vi "ArmGetStatus.vi"(0 "Pivot Ref":T1={"DeviceStatus"={"status"=FALSE, "code"=0, "source"=""}, "Type"=enum."PWM", "PWM"={"PWM Channel"=enum."PWM 1", "DeadBand"={"Name"="", "maxPositivePwm"=0, "minPositivePwm"=0, "centerPwm"=0, "maxNegativePwm"=0, "minNegativePwm"=0, "angularRange"=0}}, "CAN"={"Device Number"=0, "Control Mode"=enum."Percent VBus", "Semaphore"=refnum, "Max Vout"=12.0, "TalonSRX Control Mode"=enum."Percent VBus"}, "Invert"=FALSE, "TransformRef"=refnum, "InvTransformRef"=refnum}, 5 "ExtensionRef":T1={"DeviceStatus"={"status"=FALSE, "code"=0, "source"=""}, "Type"=enum."PWM", "PWM"={"PWM Channel"=enum."PWM 1", "DeadBand"={"Name"="", "maxPositivePwm"=0, "minPositivePwm"=0, "centerPwm"=0, "maxNegativePwm"=0, "minNegativePwm"=0, "angularRange"=0}}, "CAN"={"Device Number"=0, "Control Mode"=enum."Percent VBus", "Semaphore"=refnum, "Max Vout"=12.0, "TalonSRX Control Mode"=enum."Percent VBus"}, "Invert"=FALSE, "TransformRef"=refnum, "InvTransformRef"=refnum}, 7 "Wrist Ref":T1={"DeviceStatus"={"status"=FALSE, "code"=0, "source"=""}, "Type"=enum."PWM", "PWM"={"PWM Channel"=enum."PWM 1", "DeadBand"={"Name"="", "maxPositivePwm"=0, "minPositivePwm"=0, "centerPwm"=0, "maxNegativePwm"=0, "minNegativePwm"=0, "angularRange"=0}}, "CAN"={"Device Number"=0, "Control Mode"=enum."Percent VBus", "Semaphore"=refnum, "Max Vout"=12.0, "TalonSRX Control Mode"=enum."Percent VBus"}, "Invert"=FALSE, "TransformRef"=refnum, "InvTransformRef"=refnum}, 11 "error in (no error)":errorcluster) -> (1 "Pivot Ref out":T1={"DeviceStatus"={"status"=FALSE, "code"=0, "source"=""}, "Type"=enum."PWM", "PWM"={"PWM Channel"=enum."Invalid", "DeadBand"={"Name"="", "maxPositivePwm"=0, "minPositivePwm"=0, "centerPwm"=0, "maxNegativePwm"=0, "minNegativePwm"=0, "angularRange"=0}}, "CAN"={"Device Number"=0, "Control Mode"=enum."Percent VBus", "Semaphore"=refnum, "Max Vout"=12.0, "TalonSRX Control Mode"=enum."Percent VBus"}, "Invert"=FALSE, "TransformRef"=refnum, "InvTransformRef"=refnum}, 2 "Extension Ref out":T1={"DeviceStatus"={"status"=FALSE, "code"=0, "source"=""}, "Type"=enum."PWM", "PWM"={"PWM Channel"=enum."Invalid", "DeadBand"={"Name"="", "maxPositivePwm"=0, "minPositivePwm"=0, "centerPwm"=0, "maxNegativePwm"=0, "minNegativePwm"=0, "angularRange"=0}}, "CAN"={"Device Number"=0, "Control Mode"=enum."Percent VBus", "Semaphore"=refnum, "Max Vout"=12.0, "TalonSRX Control Mode"=enum."Percent VBus"}, "Invert"=FALSE, "TransformRef"=refnum, "InvTransformRef"=refnum}, 3 "Wrist Ref out":T1={"DeviceStatus"={"status"=FALSE, "code"=0, "source"=""}, "Type"=enum."PWM", "PWM"={"PWM Channel"=enum."Invalid", "DeadBand"={"Name"="", "maxPositivePwm"=0, "minPositivePwm"=0, "centerPwm"=0, "maxNegativePwm"=0, "minNegativePwm"=0, "angularRange"=0}}, "CAN"={"Device Number"=0, "Control Mode"=enum."Percent VBus", "Semaphore"=refnum, "Max Vout"=12.0, "TalonSRX Control Mode"=enum."Percent VBus"}, "Invert"=FALSE, "TransformRef"=refnum, "InvTransformRef"=refnum}, 4 "Pivot angle (rad)":dbl(knob) scale=3.1416..-3.1416, 6 "Extension (in.)":dbl, 8 "Wrist angle (rad, relative to ground)":dbl(knob) scale=3.1416..-3.1416, 12 "Wrist X":dbl, 14 "Wrist Y":dbl, 15 "error out":errorcluster)   [LabVIEW 2015]
uses:
  <vilib>/Rock Robotics/WPI/MotorControl/WPI_MotorControlDeviceRef.ctl
  <vilib>/Rock Robotics/WPI/MotorControl/WPI_MotorControlType.ctl
  <vilib>/Rock Robotics/SystemInterfaces/DIO/FPGA_DIOPWMChannel.ctl
  <vilib>/Rock Robotics/WPI/PWM/WPI_PWMDeadband.ctl
  <vilib>/Rock Robotics/WPI/CAN/Jaguar/SubVIs/WPI_CANJaguar_ControlMode.ctl
  <vilib>/Rock Robotics/WPI/CAN/TalonSRX/WPI_CANTalonSRX_APIControlMode.ctl
  <vilib>/Rock Robotics/WPI/PWM/WPI_PWMTransform_ConPane.ctl
  Robot Global Data.vi
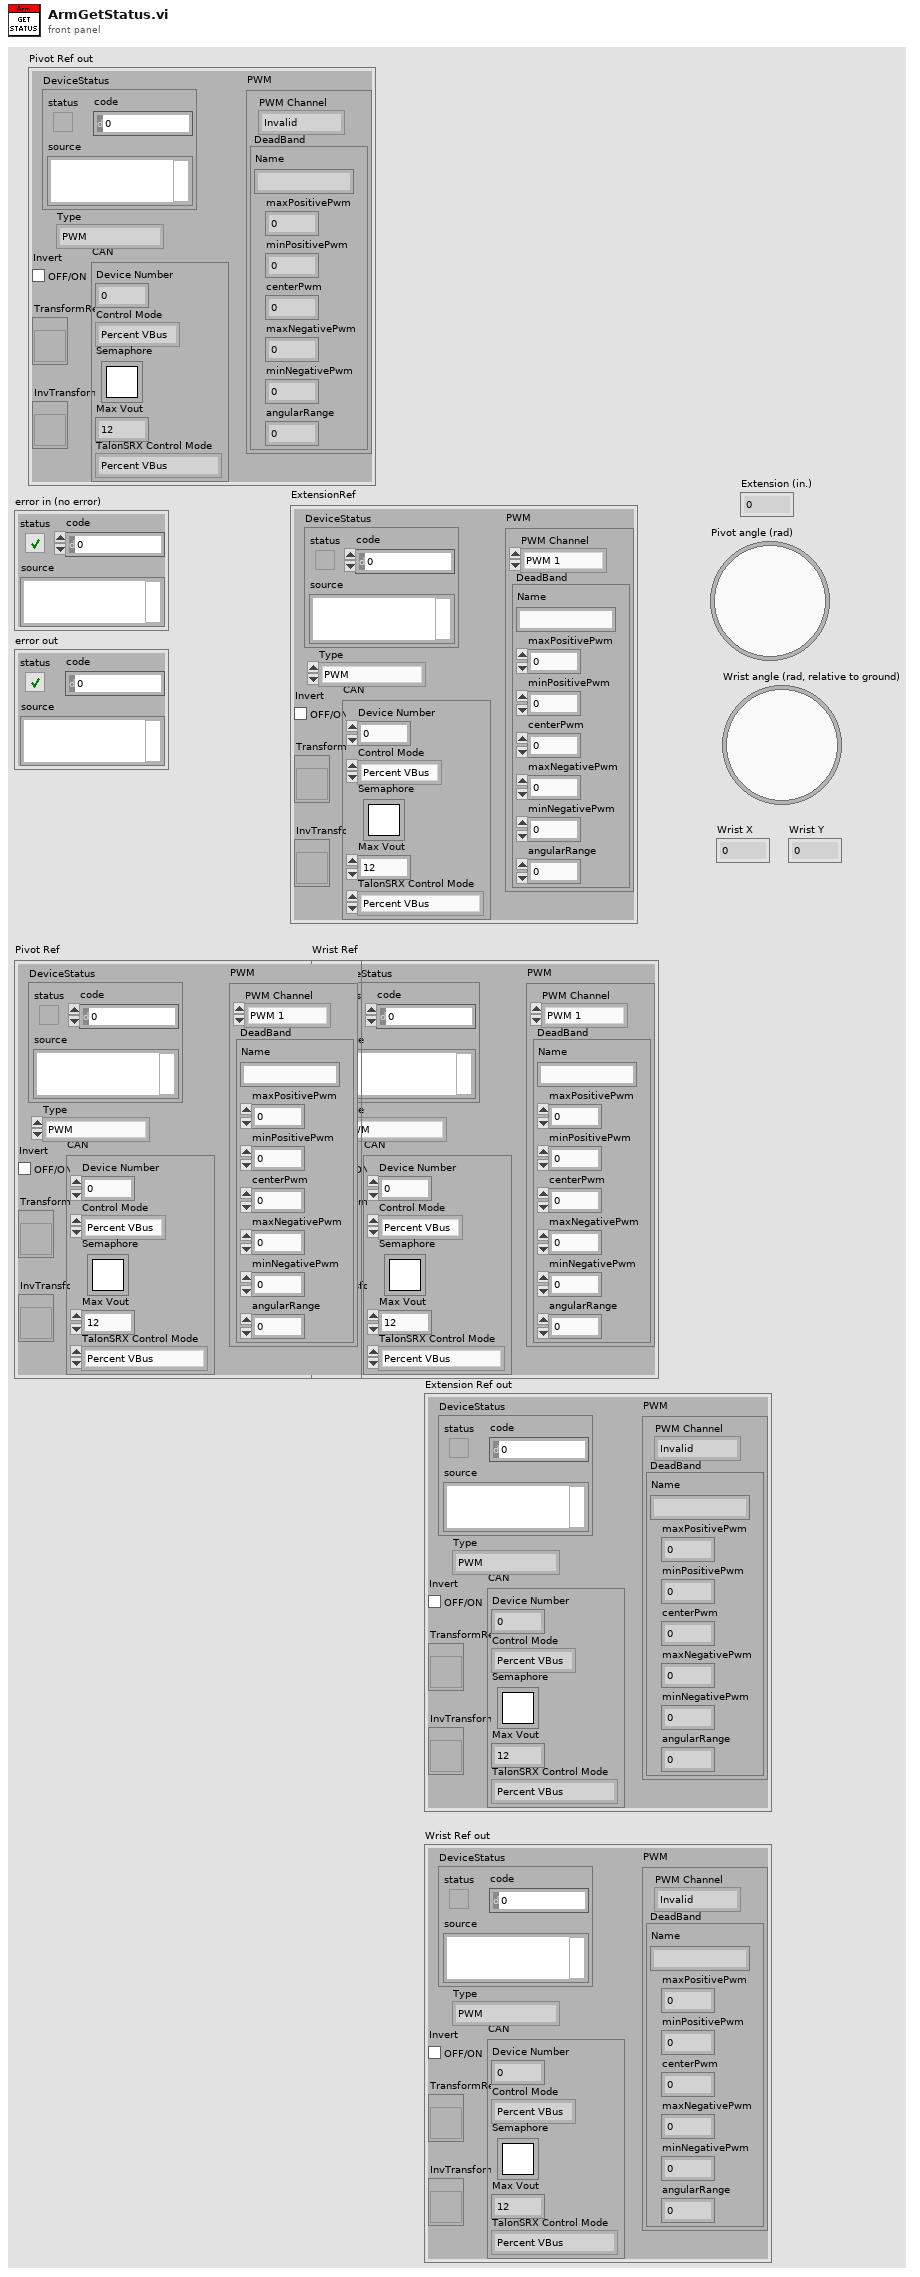
[diagram p1: front panel]
types:
  T1 = typedef "WPI_MotorControlDeviceRef.ctl" = cluster{"DeviceStatus":errorcluster, "Type":T2, "PWM":cluster{"PWM Channel":T3, "DeadBand":T4}, "CAN":cluster{"Device Number":u8, "Control Mode":T5, "Semaphore":T6, "Max Vout":dbl, "TalonSRX Control Mode":T7}, "Invert":bool, "TransformRef":T8, "InvTransformRef":T8}
  T2 = typedef "WPI_MotorControlType.ctl" = enum16{"PWM", "CAN", "CANTalonSRX"}
  T3 = typedef "FPGA_DIOPWMChannel.ctl" = enum8{"PWM 0", "PWM 1", "PWM 2", "PWM 3", "PWM 4", "PWM 5", "PWM 6", "PWM 7", "PWM 8", "PWM 9", "PWM MXP 0", "PWM MXP 1", "PWM MXP 2", "PWM MXP 3", "PWM MXP 4", "PWM MXP 5", "PWM MXP 6", "PWM MXP 7", "PWM MXP 8", "PWM MXP 9", "Invalid"}
  T4 = typedef "WPI_PWMDeadband.ctl" = cluster{"Name":string, "maxPositivePwm":i32, "minPositivePwm":i32, "centerPwm":i32, "maxNegativePwm":i32, "minNegativePwm":i32, "angularRange":u16}
  T5 = typedef "WPI_CANJaguar_ControlMode.ctl" = enum8{"Percent VBus", "Current", "Speed", "Position", "Voltage"}
  T6 = typedef "Semaphore RefNum" = refnum<k1>
  T7 = typedef "WPI_CANTalonSRX_APIControlMode.ctl" = enum8{"Percent VBus", "Speed", "Position", "Slave", "Unchanged / Invalid"}
  T8 = typedef "WPI_PWMTransform_ConPane.ctl" = refnum<vi>
  T9 = typedef "WPI_CANTalonSRX_GlobalStatus.ctl" = cluster{"Applied Throttle":dbl, "Module Enabled":bool, "CAN Error":errorcluster, "Closed Loop Error":dbl, "Forward Limit Switch Closed":bool, "Reverse Limit Switch Closed":bool, "Sensor Position":dbl, "Sensor Velocity":dbl, "Current":dbl, "Sticky Fault - Over Temp":bool, "Sticky Fault - Under Voltage":bool, "Sticky Fault - Forward Limit":bool, "Sticky Fault - Reverse Limit":bool, "Sticky Fault - Forward Soft Limit":bool, "Sticky Fault - Reverse Soft Limit":bool, "Brake is Enabled":bool, "Encoder Position":dbl, "Encoder Velocity":dbl, "Encoder Index Count":dbl, "Encoder A Pin State":bool, "Encoder B Pin State":bool, "Encoder Index Pin State":bool, "Analog In":dbl, "Analog In Velocity":dbl, "Temperature (C)":dbl, "Battery Voltage":dbl}
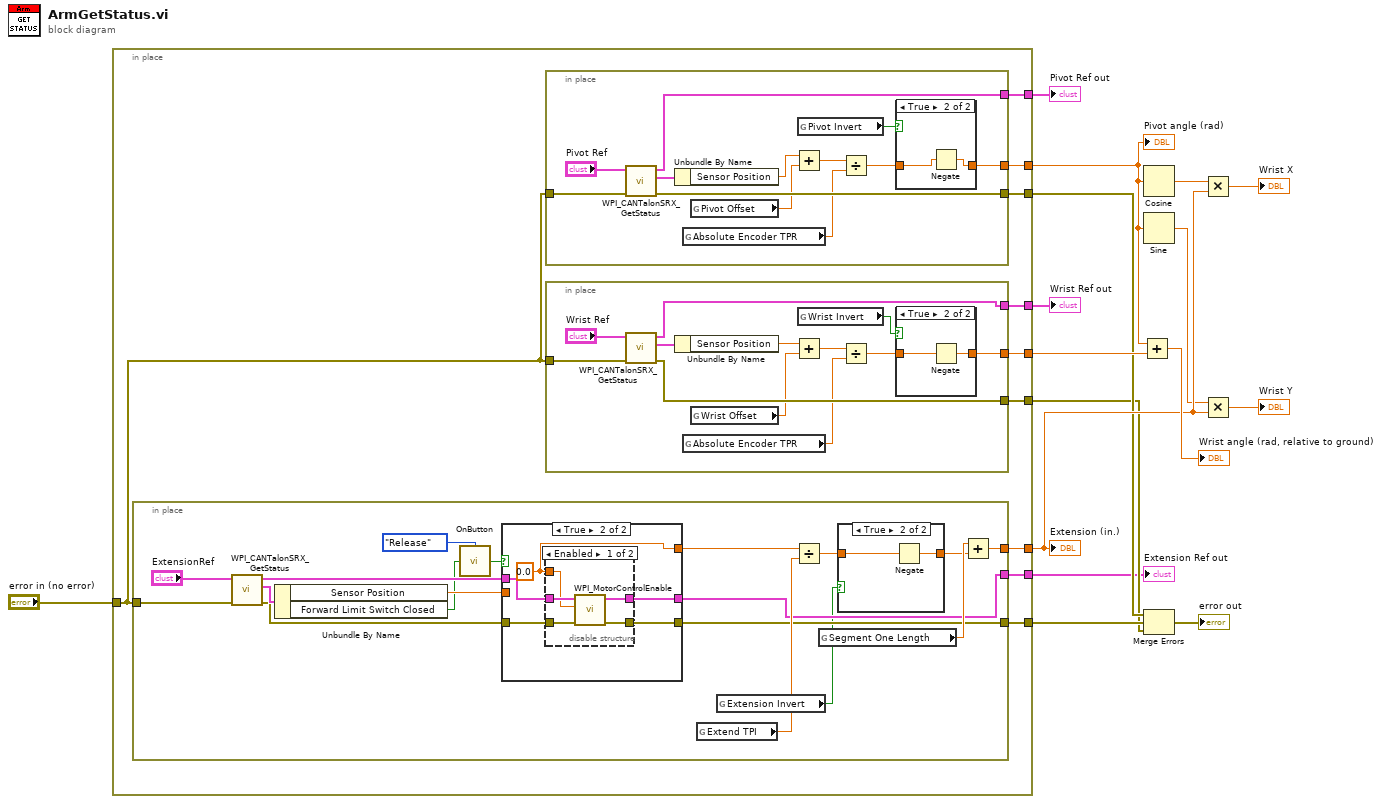
[diagram p0: block diagram]
diagram:
  n1 = in-place {
    in-place-border: "error in (no error)" -> [w26]
    in-place-border: [w25] -> w11
    in-place-border: [w24] -> w2
    in-place-border: [w23] -> w6
    in-place-border: [w22] -> w3
    in-place-border: [w21] -> w7
    in-place-border: [w18] -> w15
    in-place-border: [w17] -> w12
    in-place-border: [w20] -> w1
    in-place-border: [w19] -> w5
    n2 = in-place {
      in-place-border: w26 -> [w45]
      in-place-border: [w57] -> w25
      in-place-border: [w51] -> w24
      in-place-border: [w52] -> w23
      n3 = call <vilib>:"WPI_CANTalonSRX_GetStatus.vi"("error in (no error)"=w45, "CAN Talon SRX Ref"="ExtensionRef") -> ("error out"=w54:errorcluster, "Talon SRX Status"=w59:T9, "CAN Talon SRX Ref"=w53:T1)  [unwired: 7 in]
      n4 = Unbundle By Name(w59) -> ("Sensor Position"=w49:dbl, "Forward Limit Switch Closed"=w47:bool)
      n5 = call "OnButton.vi"("Button"=w47, "Mode"=enum16{"Press", "Release", "Both"}."Release") -> ("Value"=w46:bool)
      n6 = case shown="True" w46 {
        tunnel: w54 -> [w63 w70]
        tunnel: w53 -> [w64 w69]
        tunnel: [w63 w68] -> w52
        tunnel: [w64 w67] -> w51
        tunnel: [w65 w66] -> w50
        tunnel: w49 -> [w65 _]
        frame False {
        }
        frame True {
          w66 = 0.0 ("Encoder Initial Position")
          n7 = disable-structure shown="Enabled" {
            disable-tunnel: w70 -> [w75 w76]
            disable-tunnel: w69 -> [w74 w77]
            disable-tunnel: [w73 w76] -> w68
            disable-tunnel: [w72 w77] -> w67
            disable-tunnel: w66 -> [w71 _]
            frame Enabled {
              n8 = call <vilib>:"WPI_MotorControlEnable.vi"("error in (no error)"=w75, "Encoder Initial Position"=w71, "CAN Jaguar Ref"=w74) -> ("error out"=w73:errorcluster, "CAN Jaguar Ref"=w72:T1)  [unwired: 7 in]
            }
            frame Disabled {
            }
          }
        }
      }
      n9 = global read "Robot Global Data.vi" "Extend TPI"() -> (w58:dbl)
      n10 = global read "Robot Global Data.vi" "Extension Invert"() -> (w42:bool)
      n11 = Divide(x=w50, y=w58) -> (x/y=w56:dbl)
      n12 = global read "Robot Global Data.vi" "Segment One Length"() -> (w55:dbl)
      n13 = case shown="True" w42 {
        tunnel: w56 -> [w60 w62]
        tunnel: [w60 w61] -> w43
        frame False {
        }
        frame True {
          n14 = Negate(x=w62) -> (-x=w61:dbl)
        }
      }
      n15 = Add(x=w55, y=w43) -> (x+y=w57:dbl)
    }
    n16 = in-place {
      in-place-border: w26 -> [w81]
      in-place-border: [w85] -> w22
      in-place-border: [w89] -> w21
      in-place-border: [w79] -> w17
      n17 = call <vilib>:"WPI_CANTalonSRX_GetStatus.vi"("error in (no error)"=w81, "CAN Talon SRX Ref"="Pivot Ref") -> ("error out"=w89:errorcluster, "Talon SRX Status"=w88:T9, "CAN Talon SRX Ref"=w85:T1)  [unwired: 7 in]
      n18 = Unbundle By Name(w88) -> ("Sensor Position"=w84:dbl)
      n19 = global read "Robot Global Data.vi" "Absolute Encoder TPR"() -> (w87:dbl)
      n20 = global read "Robot Global Data.vi" "Pivot Offset"() -> (w86:dbl)
      n21 = Add(x=w84, y=w86) -> (x+y=w83:dbl)
      n22 = global read "Robot Global Data.vi" "Pivot Invert"() -> (w78:bool)
      n23 = Divide(x=w83, y=w87) -> (x/y=w82:dbl)
      n24 = case shown="True" w78 {
        tunnel: w82 -> [w90 w92]
        tunnel: [w90 w91] -> w79
        frame False {
        }
        frame True {
          n25 = Negate(x=w92) -> (-x=w91:dbl)
        }
      }
    }
    n26 = in-place {
      in-place-border: w26 -> [w38]
      in-place-border: [w36] -> w20
      in-place-border: [w35] -> w19
      in-place-border: [w34] -> w18
      n27 = call <vilib>:"WPI_CANTalonSRX_GetStatus.vi"("error in (no error)"=w38, "CAN Talon SRX Ref"="Wrist Ref") -> ("error out"=w35:errorcluster, "Talon SRX Status"=w32:T9, "CAN Talon SRX Ref"=w36:T1)  [unwired: 7 in]
      n28 = Unbundle By Name(w32) -> ("Sensor Position"=w29:dbl)
      n29 = global read "Robot Global Data.vi" "Absolute Encoder TPR"() -> (w31:dbl)
      n30 = global read "Robot Global Data.vi" "Wrist Offset"() -> (w30:dbl)
      n31 = Add(x=w29, y=w30) -> (x+y=w28:dbl)
      n32 = global read "Robot Global Data.vi" "Wrist Invert"() -> (w33:bool)
      n33 = Divide(x=w28, y=w31) -> (x/y=w37:dbl)
      n34 = case shown="True" w33 {
        tunnel: w37 -> [w39 w41]
        tunnel: [w39 w40] -> w34
        frame False {
        }
        frame True {
          n35 = Negate(x=w41) -> (-x=w40:dbl)
        }
      }
    }
  }
  "Extension (in.)" <- w11
  "Pivot angle (rad)" <- w12
  "Pivot Ref out" <- w3
  "Extension Ref out" <- w2
  "Wrist Ref out" <- w1
  n36 = Add(x=w12, y=w15) -> (x+y=→"Wrist angle (rad, relative to ground)":dbl)
  n37 = Cosine(x=w12) -> (cos(x)=w10:dbl)
  n38 = Sine(x=w12) -> (sin(x)=w9:dbl)
  n39 = Merge Errors(w7, w6, w5) -> (→"error out":errorcluster)
  n40 = Multiply(x=w10, y=w11) -> (x*y=→"Wrist X":dbl)
  n41 = Multiply(x=w9, y=w11) -> (x*y=→"Wrist Y":dbl)
